vi "VM_ProjetoV5.2.vi"() -> ()   [LabVIEW 2016, in "Projeto_Modbus_Finalizado.lvlib"]
uses:
  <vilib>/userdefined/High Color/IMAQdx.ctl
  <vilib>/Analysis/baseanly.llb/Mean (DBL).vi
  <vilib>/lvdsc/process/Deploy Library.vi
  <vilib>/Utility/file.llb/Read Delimited Spreadsheet (DBL).vi
  <vilib>/Utility/file.llb/Write Delimited Spreadsheet (DBL).vi
  <vilib>/lvdsc/process/Undeploy Library.vi
  Projeto_Modbus_Finalizado.lvlib
  <vilib>/vision/driver/NI_Vision_Acquisition_Software.lvlib
  <resource>/objmgr/imaqdx.rc
  <vilib>/Analysis/NI_AALBase.lvlib
  <vilib>/lvdsc/NI_DSC.lvlib
panel:
  in  "Calibração\nRobô":path=path "C:/Users/rodrigorg1/Desktop/Projeto/calibracaoRobo.csv"
  in  "Calibração\nMesa":path=path "C:/Users/rodrigorg1/Desktop/Projeto/calibracaoMesa.csv"
  out "Error Out":errorcluster
  in  "Cut Limit":dbl=55.0 format="%#_13g"
  in  "Confirma":bool
  out "Status":string
  out "Câmera Robo":T1(plugin-control)
  out "Câmera Mesa":T1(plugin-control)
  in  "Começa jogada":bool
  in  "stop":bool
  in  "Source Câmera Robo":T2="S1156978"
  in  "Source Câmera Mesa":T2="cam0"
  out "Dobrao":bool
  out "Passa Vez":bool
  out "place pos Norm":dbl[](array[numeric])
  out "pick pos Norm":dbl[](array[numeric])
  out "place angle":dbl
  out "pick angle":dbl
  # "x 91\ny 176"
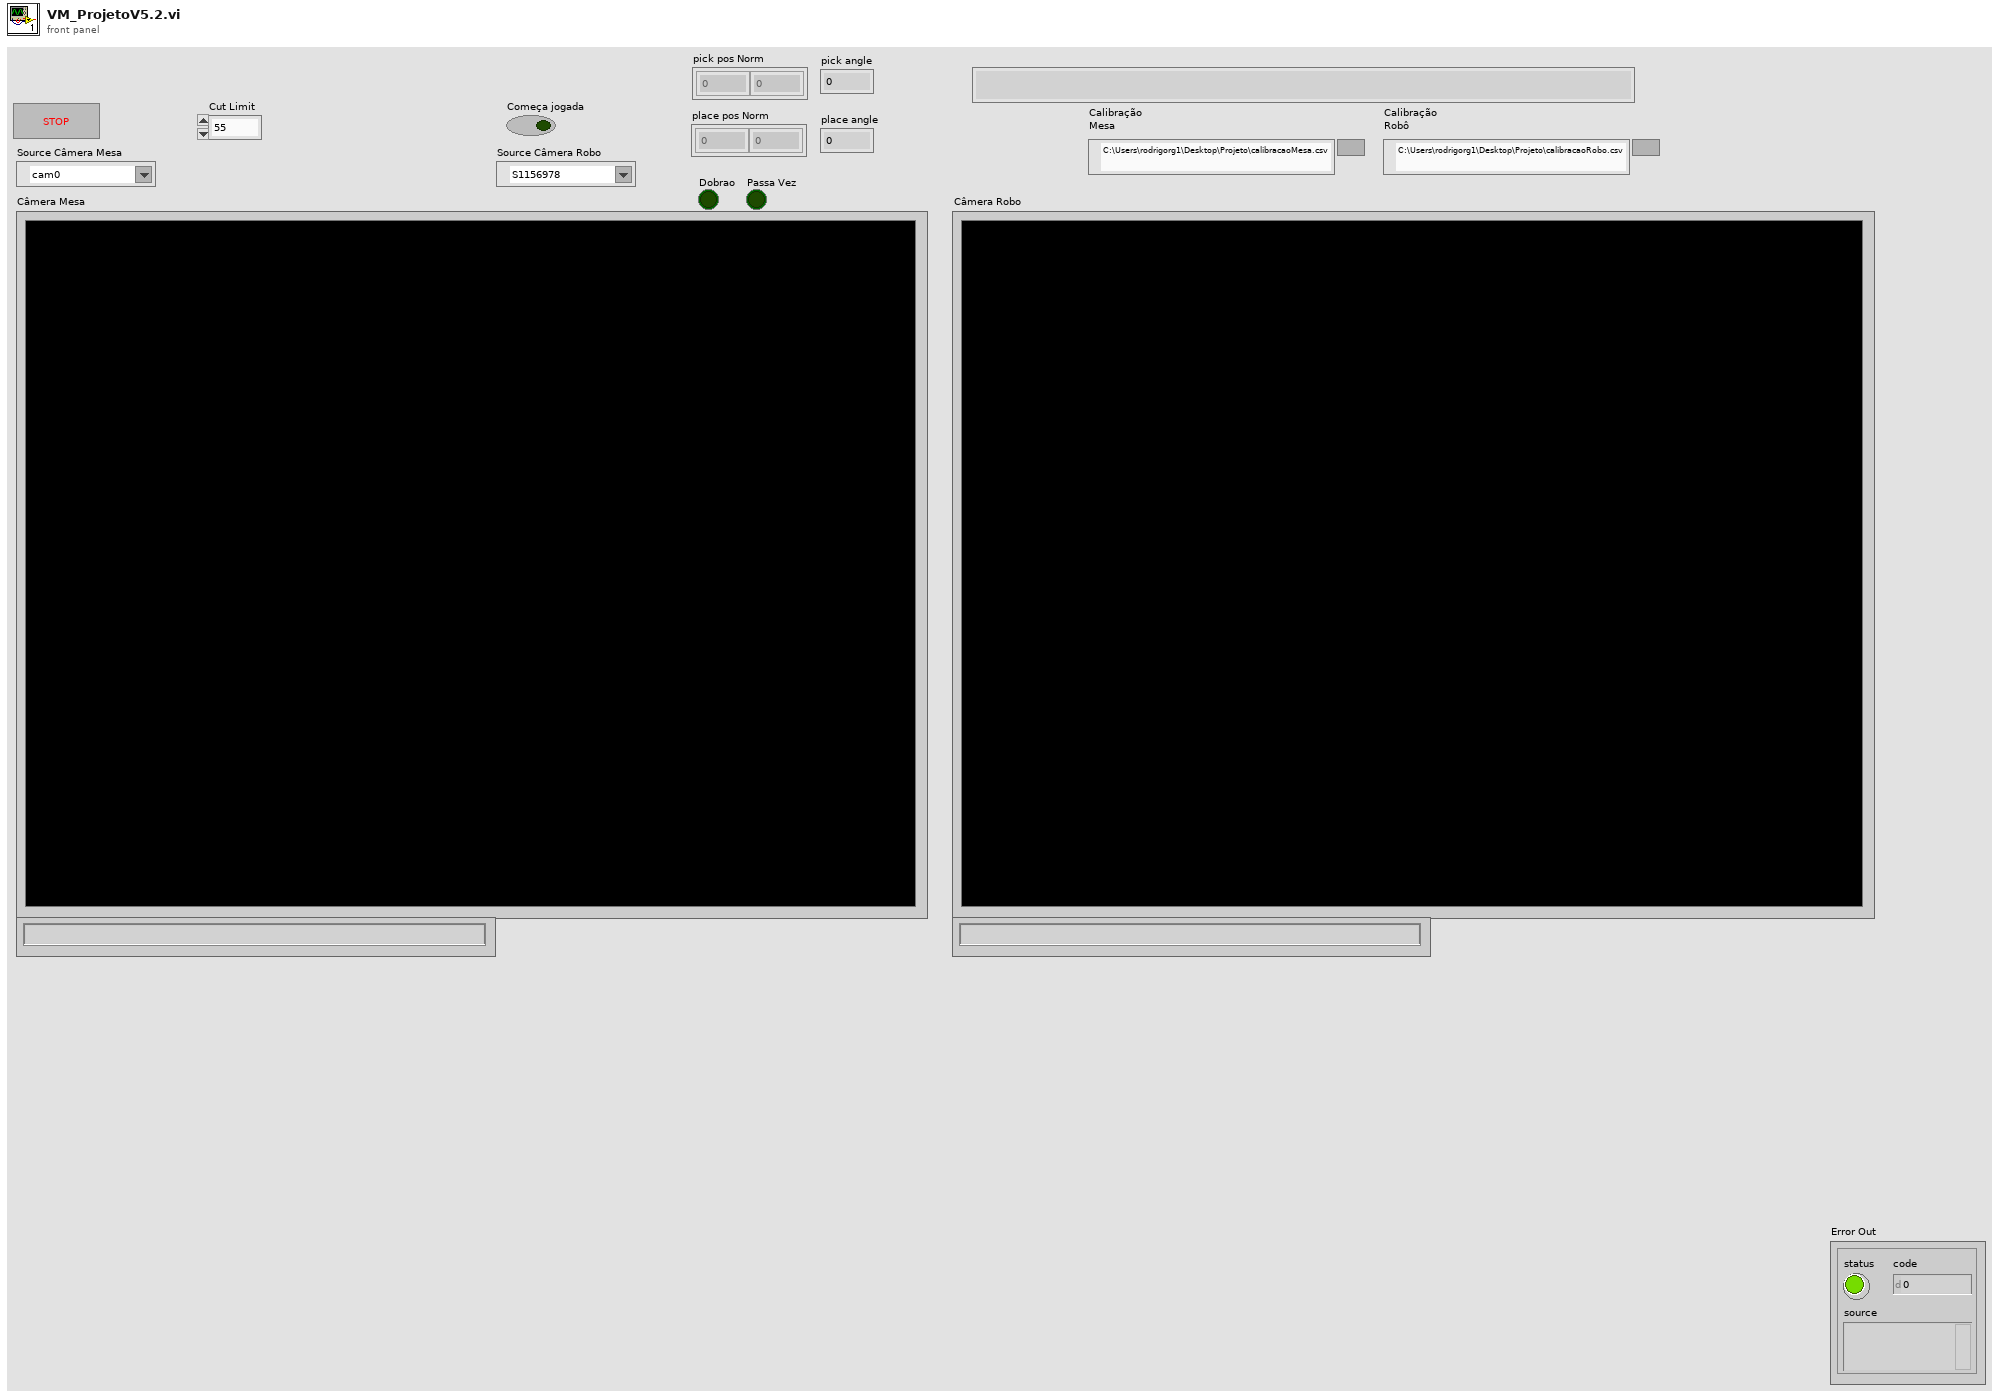
[diagram p1: front panel]
types:
  T1 = typedef "IMAQ Image.ctl" = refnum<image>
  T2 = typedef "IMAQdx.ctl" = refnum<k21>
  T3 = typedef "IMAQ Rectangle" = cluster{"Left":i32, "Top":i32, "Right":i32, "Bottom":i32, "Rotation":dbl}
  T4 = typedef "ROI Descriptor" = cluster{"Global Rectangle":i32[], "Contours":cluster{"ID":enum32{"External", "Internal"}, "Type":u32, "Coordinates":i32[]}[]}
  T5 = cluster{"Position":cluster{"x":sgl, "y":sgl}, "Angle":sgl, "Scale":sgl, "Score":sgl, "Bounding Box":cluster{"x":sgl, "y":sgl}[]}[]
  T6 = cluster{"Centro Peça":dbl[], "Centros Númeors":dbl[][], "Números":u8[], "ROI Números":T4[]}[]
  T7 = cluster{"Centro Peça":dbl[], "Centros Númeors":dbl[][], "Números":u8[], "ROI Números":T4[]}
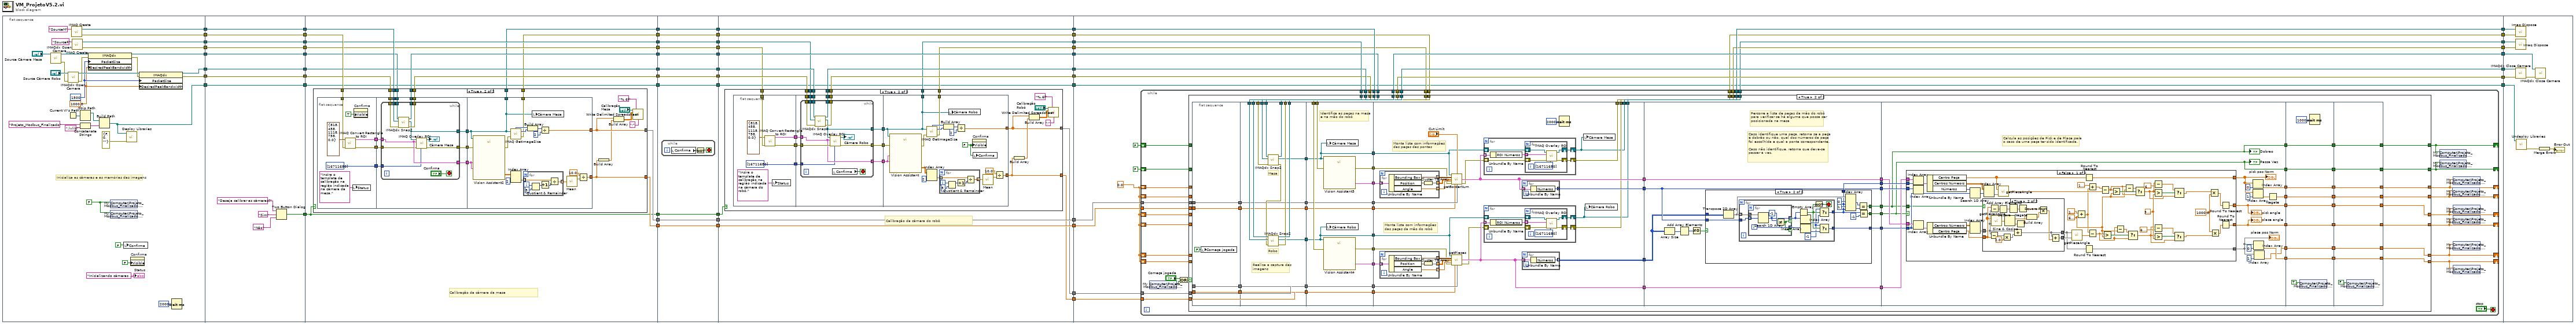
[diagram p0: block diagram]
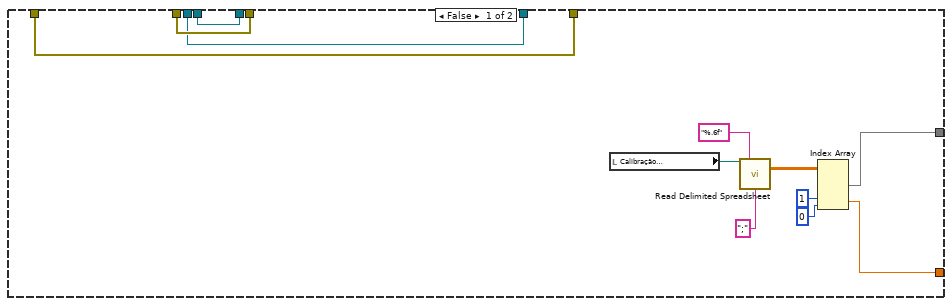
[diagram p2: hidden frame]
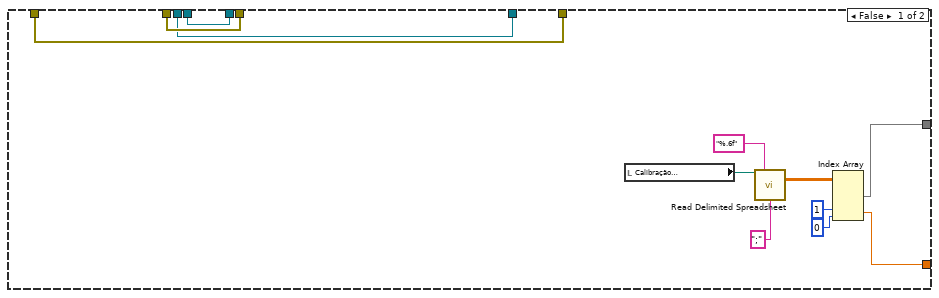
[diagram p3: hidden frame]
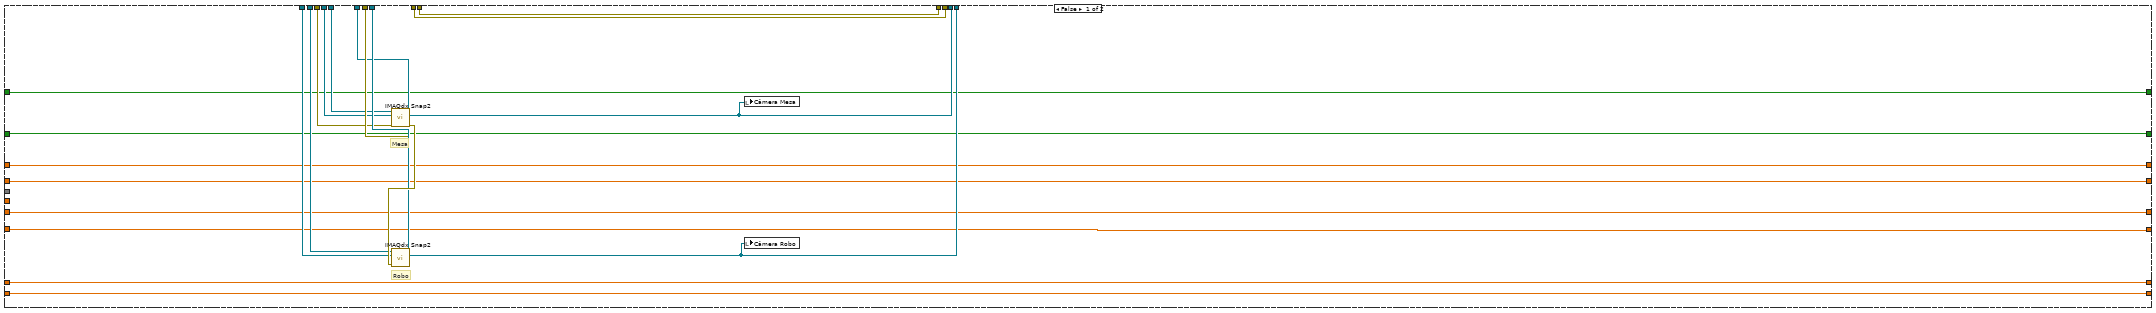
[diagram p4: hidden frame]
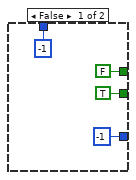
[diagram p5: hidden frame]
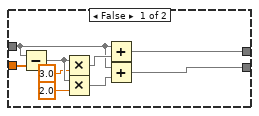
[diagram p6: hidden frame]
diagram:
  n1 = flat-sequence {
    tunnel: [w85] -> w17
    tunnel: [w84] -> w15
    tunnel: [w79] -> w13
    tunnel: [w83] -> w11
    tunnel: [w82] -> w9
    tunnel: [w78] -> w7
    tunnel: [w69] -> w5
    tunnel: [w61] -> w3
    tunnel: w17 -> [w101]
    tunnel: [w101] -> w16
    tunnel: w15 -> [w100]
    tunnel: [w100] -> w14
    tunnel: w13 -> [w99]
    tunnel: [w99] -> w12
    tunnel: w11 -> [w98]
    tunnel: [w98] -> w10
    tunnel: w9 -> [w97]
    tunnel: [w97] -> w8
    tunnel: w7 -> [w96]
    tunnel: [w96] -> w6
    tunnel: w5 -> [w95]
    tunnel: [w95] -> w4
    tunnel: w3 -> [w94]
    tunnel: [w94] -> w2
    tunnel: [w90] -> w1
    tunnel: w16 -> [w115]
    tunnel: w14 -> [w116]
    tunnel: w12 -> [w105]
    tunnel: w10 -> [w114]
    tunnel: w8 -> [w113]
    tunnel: w6 -> [w104]
    tunnel: [w109] -> w41
    tunnel: [w108] -> w39
    tunnel: [w114] -> w37
    tunnel: [w113] -> w35
    tunnel: [w112] -> w33
    tunnel: [w111] -> w31
    tunnel: w4 -> [w111]
    tunnel: [w110] -> w29
    tunnel: [w107] -> w27
    tunnel: [w106] -> w25
    tunnel: [w103] -> w20
    tunnel: w2 -> [w103]
    tunnel: [w102] -> w19
    tunnel: w1 -> [w102]
    tunnel: w41 -> [w213]
    tunnel: [w213] -> w40
    tunnel: w39 -> [w212]
    tunnel: [w212] -> w38
    tunnel: w37 -> [w211]
    tunnel: [w211] -> w36
    tunnel: w35 -> [w210]
    tunnel: [w210] -> w34
    tunnel: w33 -> [w209]
    tunnel: [w209] -> w32
    tunnel: w31 -> [w208]
    tunnel: [w208] -> w30
    tunnel: w29 -> [w207]
    tunnel: [w207] -> w28
    tunnel: w27 -> [w206]
    tunnel: [w206] -> w26
    tunnel: w25 -> [w205]
    tunnel: [w205] -> w24
    tunnel: [w204] -> w21
    tunnel: w20 -> [w204]
    tunnel: w19 -> [w203]
    tunnel: [w203] -> w18
    tunnel: w40 -> [w232]
    tunnel: [w232] -> w52
    tunnel: w38 -> [w231]
    tunnel: [w231] -> w51
    tunnel: w36 -> [w223]
    tunnel: [w222] -> w50
    tunnel: w34 -> [w221]
    tunnel: [w220] -> w49
    tunnel: w32 -> [w230]
    tunnel: [w230] -> w48
    tunnel: w30 -> [w225]
    tunnel: [w224] -> w47
    tunnel: w28 -> [w227]
    tunnel: [w226] -> w46
    tunnel: w26 -> [w229]
    tunnel: [w229] -> w45
    tunnel: w24 -> [w228]
    tunnel: [w228] -> w44
    tunnel: [w219] -> w43
    tunnel: [w218] -> w42
    tunnel: [w217] -> w22
    tunnel: w21 -> [w217]
    tunnel: w18 -> [w216]
    tunnel: [w337] -> w59
    tunnel: [w340] -> w58
    tunnel: [w334] -> w57
    tunnel: [w339] -> w56
    tunnel: [w338] -> w55
    tunnel: [w336] -> w54
    tunnel: [w335] -> w53
    tunnel: w52 -> [w333]
    tunnel: w51 -> [w332]
    tunnel: w50 -> [w331]
    tunnel: w49 -> [w330]
    tunnel: w48 -> [w329]
    tunnel: w47 -> [w328]
    tunnel: w46 -> [w327]
    tunnel: w45 -> [w325]
    tunnel: w44 -> [w326]
    tunnel: w43 -> [w323]
    tunnel: w42 -> [w324]
    tunnel: [w322] -> w23
    tunnel: w22 -> [w322]
    tunnel: w59 -> [w735]
    tunnel: w58 -> [w733]
    tunnel: w57 -> [w737]
    tunnel: w56 -> [w740]
    tunnel: w55 -> [w739]
    tunnel: w54 -> [w736]
    tunnel: w53 -> [w738]
    tunnel: w23 -> [w730]
    frame #0 {
      w60 = FALSE ("000021")
      w73 = 1000.0 ("DesiredPeakBandwidth")
      w74 = u32 1500 ("PacketSize")
      # "Inicializa as câmeras e as memórias das imagens"
      n2 = call <vilib>:"IMAQdx Open Camera.vi"("Session In"="Source Câmera Mesa") -> ("error out"=w77:errorcluster, "Session Out"=w80:T2)  [unwired: 9 in]
      n3 = Current VI's Path() -> (path=w62:path)
      n4 = call <vilib>:"IMAQdx Open Camera.vi"("error in"=w77, "Session In"="Source Câmera Robo") -> ("error out"=w76:errorcluster, "Session Out"=w81:T2)  [unwired: 8 in]
      n5 = call "IMAQ Create"("Image Name"="SourceM") -> ("New Image"=w85:T1, "error out"=w84:errorcluster)  [unwired: 4 in]
      n6 = call "IMAQ Create"("Image Name"="SourceR") -> ("New Image"=w83:T1, "error out"=w82:errorcluster)  [unwired: 4 in]
      n7 = Strip Path(path=w62) -> (stripped path=w63:path)  [unwired: 1 out]
      n8 = Concatenate Strings("Projeto_Modbus_Finalizado" ("library path"), ".lvlib" ("string")) -> (w66:string)
      n9 = property class="IMAQdx"(reference=w80, error in=w76, "PacketSize"=w74, "DesiredPeakBandwidth"=w73) -> (reference out=w79:T2, error out=w75:errorcluster)
      n10 = Build Path(base path=w63, name or relative path=w66) -> (appended path=w61:path)
      n11 = shared-variable "My Computer\\Projeto_Modbus_Finalizado.lvlib\\000021"(w60) -> ()  [unwired: 1 in, 1 out]
      n12 = shared-variable "My Computer\\Projeto_Modbus_Finalizado.lvlib\\000020"(w60) -> ()  [unwired: 1 in, 1 out]
      n13 = local write "Confirma"(FALSE ("Confirma")) -> ()
      n14 = call-poly <vilib>:"Deploy Libraries.vi"("error in (no error)"=errorcluster {"status"=FALSE, "code"=0, "source"=""}, "library path"=w61) -> ()  [unwired: 7 in, 1 out]
      n15 = property on="Confirma" class="Bool (strict)"("Visible"=FALSE) -> ()  [unwired: 2 in, 2 out]
      n16 = property class="IMAQdx"(reference=w81, error in=w75, "PacketSize"=w74, "DesiredPeakBandwidth"=w73) -> (reference out=w69:T2, error out=w78:errorcluster)
      n17 = Wait (ms)(milliseconds to wait=u32 2000) -> ()  [unwired: 1 out]
      "Status" <- "Inicializando câmeras ..." ("Status")
    }
    frame #1 {
      n18 = Two Button Dialog(message="Deseja calibrar as câmeras?", 1:"Não" ("F button name (\"Cancel\")"), 2:"Sim" ("T button name (\"OK\")")) -> (T button?=w90:bool)
    }
    frame #2 {
      # "Calibração da câmera da mesa"
      n19 = case shown="True" w102 {
        tunnel: w116 -> [w125 w143]
        tunnel: w115 -> [w126 w142]
        tunnel: [w127 w141] -> w112
        tunnel: [w128 w140] -> w110
        tunnel: [w126 w139] -> w109
        tunnel: [w125 w138] -> w108
        tunnel: [w118 w133] -> w107
        tunnel: [w117 w134] -> w106
        tunnel: w105 -> [w127 w137]
        tunnel: w104 -> [w128 w136]
        frame False {
          n20 = local read "Calibração\nMesa"() -> (w124:path)
          n21 = call-poly <vilib>:"Read Delimited Spreadsheet.vi"("file path (dialog if empty)"=w124, "format (%.3f)"="%.6f", "delimiter (\\t)"=";" ("delimiter (\\t)")) -> ("all rows"=w121:dbl[][])  [unwired: 7 in, 5 out]
          n22 = Index Array(array=w121, index (row) #2=1, index (col) #2=0) -> (element #1=w117:dbl[], element #2=w118:dbl)  [unwired: 2 in]
        }
        frame True {
          n23 = flat-sequence {
            tunnel: w143 -> [w154]
            tunnel: [w152] -> w149
            tunnel: [w151] -> w148
            tunnel: [u32[] [16711680] ("Colors (Green)")] -> w147
            tunnel: w137 -> [w167]
            tunnel: w136 -> [w166]
            tunnel: w142 -> [w165]
            tunnel: [w164] -> w141
            tunnel: [w163] -> w140
            tunnel: w149 -> [w162]
            tunnel: w148 -> [w161]
            tunnel: [w160] -> w146
            tunnel: [w159] -> w145
            tunnel: [w158] -> w144
            tunnel: w147 -> [w157]
            tunnel: w146 -> [w196]
            tunnel: w145 -> [w195]
            tunnel: [w187] -> w133
            tunnel: w144 -> [w180]
            tunnel: [w180] -> w139
            tunnel: [w182] -> w138
            tunnel: [w181] -> w134
            frame #0 {
              n24 = call "IMAQ Convert Rectangle to ROI"("error in (no error)"=w154, "Rectangle"=T3 {"Left"=818, "Top"=458, "Right"=1118, "Bottom"=758, "Rotation"=0.0}) -> ("error out"=w152:errorcluster, "ROI Descriptor"=w151:T4)  [unwired: 7 in]
              n25 = local write "Status"("Insira o template de calibração na região indicada na câmera da mesa." ("Status")) -> ()
              n26 = property on="Confirma" class="Bool (strict)"("Visible"=TRUE) -> ()  [unwired: 2 in, 2 out]
            }
            frame #1 {
              n27 = while {
                tunnel: w167 -> [w178]
                tunnel: w166 -> [w177]
                tunnel: w165 -> [w176]
                tunnel: [w175] -> w164
                tunnel: [w174] -> w163
                tunnel: w162 -> [w168]
                tunnel: w161 -> [w171]
                tunnel: [w173] -> w160
                tunnel: [w171] -> w159
                tunnel: [w169] -> w158
                tunnel: w157 -> [w170]
                stop <- "Confirma" stop-if-true
                n28 = call <vilib>:"IMAQdx Snap2.vi"("error in"=w177, "Image In"=w176, "Session In"=w178) -> ("error out"=w174:errorcluster, "Image Out"=w169:T1, "Session Out"=w175:T2)  [unwired: 6 in]
                n29 = call "IMAQ Overlay ROI"("Colors (Green)"=w170, "error in (no error)"=w168, "ROI Descriptor"=w171, "Image"=w169) -> ("error out"=w173:errorcluster, "Image Out"=→"Câmera Mesa":T1)  [unwired: 6 in]
              }
            }
            frame #2 {
              n30 = call "Vision Assistant2"("Image In"=w180, "ROI Descriptor (Adv. Straight Edge 1)"=w195, "ROI Descriptor (Copy of Adv. Straight Edge 1)"=w195, "error in"=w196) -> ("Caliper Results (Caliper 2)"=w194:sgl[][], "error out"=w188:errorcluster)  [unwired: 21 in, 1 out]
              n31 = call "IMAQ GetImageSize"("Image"=w180, "error in (no error)"=w188) -> ("Y Resolution"=w186:i32, "X Resolution"=w185:i32, "error out"=w182:errorcluster)  [unwired: 2 in]
              n32 = Index Array(array=w194, index (col)=2 ("disabled index (col)")) -> (element=w192:sgl[])  [unwired: 1 in]
              n33 = for {
                tunnel: w192 -> [w199] mode=indexing
                tunnel: [w197] -> w191 mode=indexing
                i -> [w202]
                n34 = Quotient & Remainder(x=w202, y=5) -> (x-y*floor(x/y)=w200:i32)  [unwired: 1 out]
                n35 = Increment(x=w200) -> (x+1=w198:i32)
                n36 = Divide(x=w199, y=w198) -> (x/y=w197:sgl)
              }
              n37 = Build Array(w185, w186) -> (w184:i32[])
              n38 = local write "Câmera Mesa"(w180) -> ()
              n39 = Divide(x=w184, y=2) -> (x/y=w181:dbl[])
              n40 = call-poly <vilib>:"Mean.vi"("X"=w191) -> ("mean"=w190:dbl)  [unwired: 1 out]
              n41 = Divide(x=10.0, y=w190) -> (x/y=w187:dbl)
            }
          }
          n42 = Build Array(w133) -> (w132:dbl[])
          n43 = Build Array(w134, w132) -> (w131:dbl[][])
          n44 = call-poly <vilib>:"Write Delimited Spreadsheet.vi"("file path (dialog if empty)"="Calibração\nMesa", "format (%.3f)"="%.6f", "2D data"=w131, "delimiter (\\t)"=";" ("delimiter (\\t)")) -> ()  [unwired: 10 in, 2 out]
        }
      }
    }
    frame #3 {
      n45 = while {
        stop <- w215 stop-if-true
        n46 = local read "Confirma"() -> (w214:bool)
        n47 = Not(x=w214) -> (.not. x?=w215:bool)
      }
    }
    frame #4 {
      # "Calibração da câmera do robô"
      n48 = case shown="True" w216 {
        tunnel: w227 -> [w243 w259]
        tunnel: [w243 w258] -> w226
        tunnel: w225 -> [w244 w257]
        tunnel: [w244 w256] -> w224
        tunnel: w223 -> [w242 w255]
        tunnel: [w242 w254] -> w222
        tunnel: w221 -> [w241 w253]
        tunnel: [w241 w252] -> w220
        tunnel: [w233 w246] -> w219
        tunnel: [w234 w245] -> w218
        frame False {
          n49 = local read "Calibração\nRobô"() -> (w235:path)
          n50 = call-poly <vilib>:"Read Delimited Spreadsheet.vi"("file path (dialog if empty)"=w235, "format (%.3f)"="%.6f", "delimiter (\\t)"=";" ("delimiter (\\t)")) -> ("all rows"=w238:dbl[][])  [unwired: 7 in, 5 out]
          n51 = Index Array(array=w238, index (row) #2=1, index (col) #2=0) -> (element #1=w234:dbl[], element #2=w233:dbl)  [unwired: 2 in]
        }
        frame True {
          n52 = flat-sequence {
            tunnel: w253 -> [w270]
            tunnel: [w269] -> w265
            tunnel: [w268] -> w264
            tunnel: [u32[] [16711680] ("Colors (Green)")] -> w263
            tunnel: w257 -> [w282]
            tunnel: w259 -> [w281]
            tunnel: w255 -> [w280]
            tunnel: [w279] -> w256
            tunnel: [w278] -> w258
            tunnel: w265 -> [w277]
            tunnel: w264 -> [w276]
            tunnel: [w275] -> w262
            tunnel: [w274] -> w261
            tunnel: [w273] -> w260
            tunnel: w263 -> [w272]
            tunnel: w262 -> [w312]
            tunnel: w261 -> [w311]
            tunnel: [w303] -> w246
            tunnel: w260 -> [w296]
            tunnel: [w296] -> w254
            tunnel: [w298] -> w252
            tunnel: [w297] -> w245
            frame #0 {
              n53 = call "IMAQ Convert Rectangle to ROI"("error in (no error)"=w270, "Rectangle"=T3 {"Left"=818, "Top"=458, "Right"=1118, "Bottom"=758, "Rotation"=0.0}) -> ("error out"=w269:errorcluster, "ROI Descriptor"=w268:T4)  [unwired: 7 in]
              n54 = local write "Status"("Insira o template de calibração na região indicada na câmera do robô." ("Status")) -> ()
            }
            frame #1 {
              n55 = while {
                tunnel: w282 -> [w294]
                tunnel: w281 -> [w293]
                tunnel: w280 -> [w292]
                tunnel: [w291] -> w279
                tunnel: [w290] -> w278
                tunnel: w277 -> [w289]
                tunnel: w276 -> [w287]
                tunnel: [w288] -> w275
                tunnel: [w287] -> w274
                tunnel: [w286] -> w273
                tunnel: w272 -> [w285]
                stop <- w283 stop-if-true
                n56 = call <vilib>:"IMAQdx Snap2.vi"("error in"=w293, "Image In"=w292, "Session In"=w294) -> ("error out"=w290:errorcluster, "Image Out"=w286:T1, "Session Out"=w291:T2)  [unwired: 6 in]
                n57 = call "IMAQ Overlay ROI"("Colors (Green)"=w285, "error in (no error)"=w289, "ROI Descriptor"=w287, "Image"=w286) -> ("error out"=w288:errorcluster, "Image Out"=→"Câmera Robo":T1)  [unwired: 6 in]
                n58 = local read "Confirma"() -> (w283:bool)
              }
            }
            frame #2 {
              w295 = FALSE ("Visible")
              n59 = call "Vision Assistant"("Image In"=w296, "ROI Descriptor (Adv. Straight Edge 1)"=w311, "ROI Descriptor (Copy of Adv. Straight Edge 1)"=w311, "error in"=w312) -> ("Caliper Results (Caliper 2)"=w310:sgl[][], "error out"=w304:errorcluster)  [unwired: 21 in, 1 out]
              n60 = call "IMAQ GetImageSize"("Image"=w296, "error in (no error)"=w304) -> ("Y Resolution"=w302:i32, "X Resolution"=w301:i32, "error out"=w298:errorcluster)  [unwired: 2 in]
              n61 = Index Array(array=w310, index (col)=2 ("disabled index (col)")) -> (element=w308:sgl[])  [unwired: 1 in]
              n62 = for {
                tunnel: w308 -> [w315] mode=indexing
                tunnel: [w313] -> w307 mode=indexing
                i -> [w318]
                n63 = Quotient & Remainder(x=w318, y=5) -> (x-y*floor(x/y)=w316:i32)  [unwired: 1 out]
                n64 = Increment(x=w316) -> (x+1=w314:i32)
                n65 = Divide(x=w315, y=w314) -> (x/y=w313:sgl)
              }
              n66 = Build Array(w301, w302) -> (w300:i32[])
              n67 = local write "Câmera Robo"(w296) -> ()
              n68 = Divide(x=w300, y=2) -> (x/y=w297:dbl[])
              n69 = property on="Confirma" class="Bool (strict)"("Visible"=w295) -> ()  [unwired: 2 in, 2 out]
              n70 = local write "Confirma"(w295) -> ()
              n71 = call-poly <vilib>:"Mean.vi"("X"=w307) -> ("mean"=w306:dbl)  [unwired: 1 out]
              n72 = Divide(x=10.0, y=w306) -> (x/y=w303:dbl)
            }
          }
          n73 = Build Array(w246) -> (w250:dbl[])
          n74 = Build Array(w245, w250) -> (w249:dbl[][])
          n75 = call-poly <vilib>:"Write Delimited Spreadsheet.vi"("file path (dialog if empty)"="Calibração\nRobô", "format (%.3f)"="%.6f", "2D data"=w249, "delimiter (\\t)"=";" ("delimiter (\\t)")) -> ()  [unwired: 10 in, 2 out]
        }
      }
    }
    frame #5 {
      w319 = 0.0 ("Numeric")
      n76 = while {
        tunnel: w329 -> [w378]
        tunnel: w333 -> [w377]
        tunnel: w331 -> [w376]
        tunnel: w328 -> [w375]
        tunnel: w327 -> [w374]
        tunnel: [w373] -> w340
        tunnel: [w372] -> w339
        tunnel: [w371] -> w338
        tunnel: w332 -> [w370]
        tunnel: w330 -> [w369]
        tunnel: [w368] -> w337
        tunnel: [w367] -> w334
        tunnel: [w365] -> w336
        tunnel: [w364] -> w335
        tunnel: w326 -> [w363]
        tunnel: w325 -> [w362]
        tunnel: w324 -> [w361]
        tunnel: w323 -> [w360]
        shift-right: [w356] -> _
        shift-left: FALSE -> [w347]
        shift-right: [w355] -> _
        shift-left: FALSE -> [w348]
        shift-right: [w354] -> _
        shift-left: w319 -> [w346]
        shift-right: [w353] -> _
        shift-left: w319 -> [w345]
        shift-right: [w352] -> _
        shift-left: w319 -> [w344]
        shift-right: [w351] -> _
        shift-left: w319 -> [w343]
        shift-right: [w350] -> _
        shift-left: w319 -> [w342]
        shift-right: [w349] -> _
        shift-left: w319 -> [w341]
        stop <- "stop" stop-if-true
        n77 = shared-variable "My Computer\\Projeto_Modbus_Finalizado.lvlib\\000022"() -> (w357:bool)  [unwired: 1 in, 1 out]
        n78 = Or(x="Começa jogada", y=w357) -> (x .or. y?=w359:bool)
        n79 = case shown="True" w359 {
          tunnel: w378 -> [w390 w472]
          tunnel: w377 -> [w389 w471]
          tunnel: w376 -> [w396 w470]
          tunnel: w375 -> [w395 w469]
          tunnel: w374 -> [w392 w468]
          tunnel: [w391 w467] -> w373
          tunnel: [w394 w466] -> w372
          tunnel: [w393 w465] -> w371
          tunnel: w370 -> [w399 w463]
          tunnel: w369 -> [w398 w461]
          tunnel: [w388 w429] -> w368
          tunnel: [w387 w430] -> w367
          tunnel: [w399 w427] -> w365
          tunnel: [w398 w428] -> w364
          tunnel: w363 -> [_ w416]
          tunnel: w362 -> [_ w443]
          tunnel: w361 -> [_ w418]
          tunnel: w360 -> [_ w417]
          tunnel: [w384 w426] -> w354
          tunnel: [w382 w425] -> w353
          tunnel: [w383 w424] -> w352
          tunnel: [w381 w423] -> w351
          tunnel: [w380 w422] -> w350
          tunnel: [w379 w421] -> w349
          tunnel: [w385 w420] -> w356
          tunnel: [w386 w419] -> w355
          tunnel: w348 -> [w386 _]
          tunnel: w347 -> [w385 _]
          tunnel: w346 -> [w384 _]
          tunnel: w345 -> [w382 _]
          tunnel: w344 -> [w383 _]
          tunnel: w343 -> [w381 _]
          tunnel: w342 -> [w380 _]
          tunnel: w341 -> [w379 _]
          frame False {
            # "Robo"
            # "Mesa"
            n80 = call <vilib>:"IMAQdx Snap2.vi"("error in"=w392, "Image In"=w389, "Session In"=w390) -> ("error out"=w397:errorcluster, "Image Out"=w388:T1, "Session Out"=w391:T2)  [unwired: 6 in]
            n81 = call <vilib>:"IMAQdx Snap2.vi"("error in"=w397, "Image In"=w396, "Session In"=w395) -> ("error out"=w393:errorcluster, "Image Out"=w387:T1, "Session Out"=w394:T2)  [unwired: 6 in]
            n82 = local write "Câmera Mesa"(w388) -> ()
            n83 = local write "Câmera Robo"(w387) -> ()
          }
          frame True {
            n84 = flat-sequence {
              tunnel: w417 -> [w474]
              tunnel: w418 -> [w475]
              tunnel: w443 -> [w476]
              tunnel: w416 -> [w477]
              tunnel: [w477] -> w434
              tunnel: [w476] -> w433
              tunnel: [w475] -> w432
              tunnel: [w474] -> w431
              tunnel: w472 -> [w492]
              tunnel: w471 -> [w491]
              tunnel: w470 -> [w490]
              tunnel: w469 -> [w489]
              tunnel: w468 -> [w483]
              tunnel: [w488] -> w467
              tunnel: [w487] -> w466
              tunnel: [w486] -> w465
              tunnel: [w485] -> w464
              tunnel: [w484] -> w462
              tunnel: [w481] -> w441
              tunnel: [w480] -> w439
              tunnel: [w479] -> w437
              tunnel: [w478] -> w436
              tunnel: w434 -> [w481]
              tunnel: w433 -> [w480]
              tunnel: w432 -> [w479]
              tunnel: w431 -> [w478]
              tunnel: w464 -> [w494]
              tunnel: w463 -> [w504]
              tunnel: w462 -> [w493]
              tunnel: w461 -> [w503]
              tunnel: [w502] -> w460
              tunnel: [w501] -> w459
              tunnel: [w493] -> w458
              tunnel: [w494] -> w457
              tunnel: [w500] -> w456
              tunnel: [w499] -> w455
              tunnel: [w498] -> w442
              tunnel: w441 -> [w498]
              tunnel: [w497] -> w440
              tunnel: w439 -> [w497]
              tunnel: [w496] -> w438
              tunnel: w437 -> [w496]
              tunnel: w436 -> [w495]
              tunnel: [w495] -> w435
              tunnel: w460 -> [w532]
              tunnel: w459 -> [w531]
              tunnel: w458 -> [w506]
              tunnel: w457 -> [w507]
              tunnel: w456 -> [w527]
              tunnel: w455 -> [w523]
              tunnel: [w522] -> w454
              tunnel: [w521] -> w453
              tunnel: [w515] -> w452
              tunnel: [w513] -> w451
              tunnel: w442 -> [w520]
              tunnel: w440 -> [w519]
              tunnel: w438 -> [w518]
              tunnel: w435 -> [w517]
              tunnel: [w508] -> w430
              tunnel: [w511] -> w428
              tunnel: [w509] -> w429
              tunnel: [w510] -> w427
              tunnel: w454 -> [w575]
              tunnel: w453 -> [w574]
              tunnel: w452 -> [w581]
              tunnel: w451 -> [w577]
              tunnel: [w581] -> w450
              tunnel: [w580] -> w449
              tunnel: [w579] -> w448
              tunnel: [w578] -> w447
              tunnel: [w577] -> w446
              tunnel: [w576] -> w445
              tunnel: [w575] -> w444
              tunnel: w450 -> [w631]
              tunnel: w449 -> [w621]
              tunnel: w448 -> [w622]
              tunnel: w447 -> [w634]
              tunnel: w446 -> [w630]
              tunnel: w445 -> [w633]
              tunnel: w444 -> [w632]
              tunnel: [w623] -> w415
              tunnel: [w615] -> w414
              tunnel: [w620] -> w413
              tunnel: [w619] -> w412
              tunnel: [w617] -> w411
              tunnel: [w618] -> w410
              tunnel: [w622] -> w409
              tunnel: [w621] -> w408
              tunnel: w415 -> [w720]
              tunnel: w414 -> [w719]
              tunnel: w413 -> [w718]
              tunnel: w412 -> [w717]
              tunnel: w411 -> [w716]
              tunnel: w410 -> [w715]
              tunnel: w409 -> [w714]
              tunnel: w408 -> [w713]
              tunnel: [w720] -> w407
              tunnel: [w719] -> w406
              tunnel: [w718] -> w405
              tunnel: [w717] -> w404
              tunnel: [w716] -> w403
              tunnel: [w715] -> w402
              tunnel: [w714] -> w401
              tunnel: [w713] -> w400
              tunnel: [w722] -> w419
              tunnel: [w723] -> w420
              tunnel: [w724] -> w421
              tunnel: [w725] -> w422
              tunnel: [w726] -> w423
              tunnel: [w727] -> w424
              tunnel: [w728] -> w425
              tunnel: [w729] -> w426
              tunnel: w407 -> [w729]
              tunnel: w406 -> [w728]
              tunnel: w405 -> [w727]
              tunnel: w404 -> [w726]
              tunnel: w403 -> [w725]
              tunnel: w402 -> [w724]
              tunnel: w401 -> [w723]
              tunnel: w400 -> [w722]
              frame #0 {
                n85 = local write "Começa jogada"(FALSE ("Começa jogada")) -> ()
              }
              frame #1 {
                # "Realiza a captura das\nimagens"
                # "Robo"
                # "Mesa"
                n86 = call <vilib>:"IMAQdx Snap2.vi"("error in"=w483, "Image In"=w491, "Session In"=w492) -> ("error out"=w482:errorcluster, "Image Out"=w485:T1, "Session Out"=w488:T2)  [unwired: 6 in]
                n87 = call <vilib>:"IMAQdx Snap2.vi"("error in"=w482, "Image In"=w490, "Session In"=w489) -> ("error out"=w486:errorcluster, "Image Out"=w484:T1, "Session Out"=w487:T2)  [unwired: 6 in]
              }
              frame #2 {
                # "Identifica as peças na mesa\ne na mão do robô"
                n88 = call "Vision Assistant3"("Image In"=w494, "error in"=w504) -> ("Matches (Pattern Matching 1)"=w501:T5, "error out"=w500:errorcluster)  [unwired: 23 in, 1 out]
                n89 = call "Vision Assistant4"("Image In"=w493, "error in"=w503) -> ("Matches (Pattern Matching 1)"=w502:T5, "error out"=w499:errorcluster)  [unwired: 23 in, 1 out]
                n90 = local write "Câmera Mesa"(w494) -> ()
                n91 = local write "Câmera Robo"(w493) -> ()
              }
              frame #3 {
                # "Monta lista com informações\ndas peças das pontas"
                # "Monta lista com informações\ndas peças da mão do robô"
                n92 = for {
                  tunnel: w531 -> [w565] mode=indexing
                  tunnel: [w563] -> w529 mode=indexing
                  tunnel: [w562] -> w530 mode=indexing
                  tunnel: [w561] -> w528 mode=indexing
                  n93 = Unbundle By Name(w565) -> ("Bounding Box"=w562:cluster{"x":sgl, "y":sgl}[], "Position"=w564:cluster{"x":sgl, "y":sgl}, "Angle"=w561:sgl)
                  n94 = Cluster To Array(cluster=w564) -> (array=w563:sgl[])
                }
                n95 = for {
                  tunnel: w532 -> [w570] mode=indexing
                  tunnel: [w568] -> w525 mode=indexing
                  tunnel: [w567] -> w526 mode=indexing
                  tunnel: [w566] -> w524 mode=indexing
                  n96 = Unbundle By Name(w570) -> ("Bounding Box"=w567:cluster{"x":sgl, "y":sgl}[], "Position"=w569:cluster{"x":sgl, "y":sgl}, "Angle"=w566:sgl)
                  n97 = Cluster To Array(cluster=w569) -> (array=w568:sgl[])
                }
                n98 = call "getBorderNum.vi"("Refnum in"=w507, "Cut Limit"="Cut Limit", "Bounding Box"=w530, "Position"=w529, "Angle"=w528, "error in (no error)"=w527, "Step"=w519, "Origin Pixel"=w520) -> ("Data Pieces"=w515:T6, "error out"=w514:errorcluster)  [unwired: 5 in, 1 out]
                n99 = call "getPieces.vi"("Refnum in"=w506, "Bounding Box"=w526, "Position"=w525, "Angle"=w524, "error in (no error)"=w523, "Step"=w517, "Origin Pixel"=w518) -> ("Data Pieces"=w513:T6, "error out"=w512:errorcluster)  [unwired: 6 in, 1 out]
                n100 = for {
                  tunnel: w515 -> [w550] mode=indexing
                  shift-right: [w547] -> w509
                  shift-left: w507 -> [w548]
                  shift-right: [w545] -> w510
                  shift-left: w514 -> [w546]
                  n101 = Unbundle By Name(w550) -> ("ROI Números"=w549:T4[])
                  n102 = for {
                    tunnel: w549 -> [w556] mode=indexing
                    shift-right: [w554] -> w547
                    shift-left: w548 -> [w555]
                    shift-right: [w552] -> w545
                    shift-left: w546 -> [w553]
                    n103 = call "IMAQ Overlay ROI"("Colors (Green)"=u32[] [16711680], "error in (no error)"=w553, "ROI Descriptor"=w556, "Image"=w555) -> ("error out"=w552:errorcluster, "Image Out"=w554:T1)  [unwired: 6 in]
                  }
                }
                n104 = for {
                  tunnel: w513 -> [w538] mode=indexing
                  shift-right: [w535] -> w508
                  shift-left: w506 -> [w536]
                  shift-right: [w533] -> w511
                  shift-left: w512 -> [w534]
                  n105 = Unbundle By Name(w538) -> ("ROI Números"=w537:T4[])
                  n106 = for {
                    tunnel: w537 -> [w544] mode=indexing
                    shift-right: [w542] -> w535
                    shift-left: w536 -> [w543]
                    shift-right: [w540] -> w533
                    shift-left: w534 -> [w541]
                    n107 = call "IMAQ Overlay ROI"("Colors (Green)"=u32[] [16711680], "error in (no error)"=w541, "ROI Descriptor"=w544, "Image"=w543) -> ("error out"=w540:errorcluster, "Image Out"=w542:T1)  [unwired: 6 in]
                  }
                }
                n108 = for {
                  tunnel: w515 -> [w560] mode=indexing
                  tunnel: [w559] -> w522 mode=concatenating
                  n109 = Unbundle By Name(w560) -> ("Números"=w559:u8[])
                }
                n110 = for {
                  tunnel: w513 -> [w558] mode=indexing
                  tunnel: [w557] -> w521 mode=indexing
                  n111 = Unbundle By Name(w558) -> ("Números"=w557:u8[])
                }
                n112 = Wait (ms)(milliseconds to wait=u32 2000) -> ()  [unwired: 1 out]
                n113 = local write "Câmera Mesa"(w509) -> ()
                n114 = local write "Câmera Robo"(w508) -> ()
              }
              frame #4 {
                # "Caso identifique uma peça, retorna se a peça\né dobrão ou não, qual dos números da peça\nfoi escolhida e qual a ponta correspondente.\n\nCaso não identifique, retorna que deve-se\npassar a vez."
                # "Percorre a lista de peças da mão do robô\npara verificar se há alguma que possa ser\nposicionada na mesa"
                n115 = Array Size(array=w574) -> (size(s)=w573:i32[])
                n116 = Add Array Elements(numeric array=w573) -> (sum=w572:i32)
                n117 = Not Equal To 0?(x=w572) -> (x != 0?=w571:bool)
                n118 = case shown="True" w571 {
                  tunnel: w574 -> [_ w591]
                  tunnel: [FALSE w590] -> w580
                  tunnel: [TRUE w589] -> w579
                  tunnel: [-1 ("t") w588] -> w578
                  tunnel: [-1 ("index of element") w587] -> w576
                  tunnel: w575 -> [_ w586]
                  frame False {
                  }
                  frame True {
                    n119 = Transpose 2D Array(2D array=w591) -> (transposed array=w593:u8[][])
                    n120 = for {
                      tunnel: w593 -> [w608] mode=indexing
                      tunnel: w586 -> [w607]
                      tunnel: [w599] -> w588
                      tunnel: [w598] -> w587
                      stop <- w603 stop-if-true
                      w600 = -1 ("t")
                      n121 = for {
                        tunnel: w608 -> [w614]
                        tunnel: w607 -> [w613] mode=indexing
                        tunnel: [w611] -> w605 mode=indexing if=w609
                        tunnel: [w610] -> w604 mode=indexing if=w609
                        i -> [w610]
                        n122 = Search 1D Array(1D array=w614, element=w613) -> (index of element=w611:i32)  [unwired: 1 in]
                        n123 = Not Equal?(x=w611, y=-1) -> (x != y?=w609:bool)
                      }
                      n124 = Empty Array?(array=w605) -> (empty?=w601:bool)
                      n125 = Index Array(array=w605) -> (element=w606:i32)  [unwired: 1 in]
                      n126 = Index Array(array=w604) -> (element=w602:i32)  [unwired: 1 in]
                      n127 = Not(x=w601) -> (.not. x?=w603:bool)
                      n128 = Select(t=w600, s=w601, f=w606) -> (s? t:f=w598:i32)
                      n129 = Select(t=w600, s=w601, f=w602) -> (s? t:f=w599:i32)
                    }
                    n130 = Index Array(array=w593, index (row) #1=0 ("disabled index (row)"), index (col) #1=w587, index (row) #2=1 ("disabled index (row)"), index (col) #2=w587) -> (element #1=w597:u8, element #2=w596:u8)
                    n131 = Equal?(x=w597, y=w596) -> (x = y?=w590:bool)
                    n132 = Equal?(x=w587, y=-1) -> (x = y?=w589:bool)
                  }
                }
              }
              frame #5 {
                # "Calcula as posições de Pick e de Place para\no caso de uma peça ter sido identificada."
                n133 = case shown="False" w622 {
                  tunnel: w630 -> [w680 _]
                  tunnel: w633 -> [w679 _]
                  tunnel: w634 -> [w676 _]
                  tunnel: w631 -> [w678 _]
                  tunnel: w632 -> [w668 _]
                  tunnel: w621 -> [w673 _]
                  tunnel: [w666 _] -> w628
                  tunnel: [w665 _] -> w624
                  tunnel: [w661 _] -> w619
                  tunnel: [w662 _] -> w620
                  frame False {
                    w645 = 3.141592653589793
                    w649 = 6.283185307179586
                    w667 = 1000.0
                    n134 = Index Array(array=w680, index=w679) -> (element=w681:T7)
                    n135 = Index Array(array=w668, index=w676) -> (element=w675:u8)
                    n136 = Index Array(array=w678, index=w676) -> (element=w677:T7)
                    n137 = Unbundle By Name(w681) -> ("Centro Peça"=w663:dbl[], "Centros Númeors"=w683:dbl[][], "Números"=w682:u8[])
                    n138 = Unbundle By Name(w677) -> ("Centros Númeors"=w670:dbl[][], "Centro Peça"=w669:dbl[])
                    n139 = Search 1D Array(1D array=w682, element=w675) -> (index of element=w684:i32)  [unwired: 1 in]
                    n140 = Index Array(array=w670) -> (element=w672:dbl[])  [unwired: 2 in]
                    n141 = case shown="True" w673 {
                      tunnel: w672 -> [w688 w703]
                      tunnel: w669 -> [w692 w704]
                      tunnel: [w686 w696] -> w671
                      tunnel: [w685 w695] -> w664
                      frame False {
                        n142 = Subtract(x=w688, y=w692) -> (x-y=w691:dbl[])
                        n143 = Multiply(x=w691, y=3.0) -> (x*y=w693:dbl[])
                        n144 = Multiply(x=w691, y=2.0) -> (x*y=w687:dbl[])
                        n145 = Add(x=w688, y=w693) -> (x+y=w685:dbl[])
                        n146 = Add(x=w688, y=w687) -> (x+y=w686:dbl[])
                      }
                      frame True {
                        n147 = Subtract(x=w703, y=w704) -> (x-y=w710:dbl[])
                        n148 = Subtract(x=w704, y=w703) -> (x-y=w707:dbl[])
                        n149 = call "getPieceAngle.vi"("Center Num"=w703, "Center Piece"=w704) -> ("Angle"=w702:dbl)
                        n150 = Square(x=w707) -> (x^2=w706:dbl[])
                        n151 = Multiply(x=w710, y=2.0) -> (x*y=w708:dbl[])
                        n152 = Sine & Cosine(0:w702) -> (1:w700:dbl, 2:w701:dbl)
                        n153 = Add Array Elements(numeric array=w706) -> (sum=w705:dbl)
                        n154 = Add(x=w703, y=w708) -> (x+y=w695:dbl[])
                        n155 = Negate(x=w701) -> (-x=w699:dbl)
                        n156 = Square Root(x=w705) -> (sqrt(x)=w697:dbl)
                        n157 = Build Array(w699, w700) -> (w698:dbl[])
                        n158 = Multiply(x=w697, y=w698) -> (x*y=w694:dbl[])
                        n159 = Add(x=w695, y=w694) -> (x+y=w696:dbl[])
                      }
                    }
                    n160 = Index Array(array=w683, index (row)=w684) -> (element=w674:dbl[])  [unwired: 1 in]
                    n161 = call "getPieceAngle.vi"("Center Num"=w674, "Center Piece"=w663) -> ("Angle"=w657:dbl)
                    n162 = call "getPieceAngle.vi"("Center Num"=w671, "Center Piece"=w664) -> ("Angle"=w658:dbl)
                    n163 = Add(x=1.5707963267948966, y=w649) -> (x+y=w648:dbl)
                    n164 = Round To Nearest(number=w663) -> (nearest integer value=w666:dbl[])
                    n165 = Round To Nearest(number=w664) -> (nearest integer value=w665:dbl[])
                    n166 = Add(x=1.5707963267948966, y=w648) -> (x+y=w647:dbl)
                    n167 = Subtract(x=w648, y=w658) -> (x-y=w650:dbl)
                    n168 = Subtract(x=w647, y=w657) -> (x-y=w653:dbl)
                    n169 = Greater?(x=w650, y=w649) -> (0:w655:bool)
                    n170 = Greater?(x=w653, y=w649) -> (0:w654:bool)
                    n171 = Subtract(x=w650, y=w649) -> (x-y=w651:dbl)
                    n172 = Subtract(x=w653, y=w649) -> (x-y=w652:dbl)
                    n173 = Select(t=w651, s=w655, f=w650) -> (s? t:f=w639:dbl)
                    n174 = Select(t=w652, s=w654, f=w653) -> (s? t:f=w642:dbl)
                    n175 = Subtract(x=w642, y=6.283185307179586) -> (x-y=w635:dbl)
                    n176 = Greater?(x=w642, y=w645) -> (0:w644:bool)
                    n177 = Subtract(x=w639, y=6.283185307179586) -> (x-y=w638:dbl)
                    n178 = Greater?(x=w639, y=w645) -> (0:w643:bool)
                    n179 = Select(t=w635, s=w644, f=w642) -> (s? t:f=w636:dbl)
                    n180 = Select(t=w638, s=w643, f=w639) -> (s? t:f=w637:dbl)
                    n181 = Multiply(x=w636, y=w667) -> (x*y=w660:dbl)
                    n182 = Multiply(x=w667, y=w637) -> (x*y=w659:dbl)
                    n183 = Round To Nearest(number=w660) -> (nearest integer value=w662:dbl)
                    n184 = Round To Nearest(number=w659) -> (nearest integer value=w661:dbl)
                  }
                  frame True {
                  }
                }
                "pick angle" <- w620
                "pick pos Norm" <- w628
                "place angle" <- w619
                "place pos Norm" <- w624
                n185 = Index Array(array=w628, index=0) -> (element=w623:dbl)
                n186 = Index Array(array=w628, index=1) -> (element=w616:dbl)
                n187 = Index Array(array=w624, index=0) -> (element=w618:dbl)
                n188 = Index Array(array=w624, index=1) -> (element=w617:dbl)
                n189 = Negate(x=w616) -> (-x=w615:dbl)
                "Passa Vez" <- w622
                "Dobrao" <- w621
              }
              frame #6 {
                n190 = shared-variable "My Computer\\Projeto_Modbus_Finalizado.lvlib\\000021"(TRUE ("000021")) -> ()  [unwired: 1 in, 1 out]
                n191 = Wait (ms)(milliseconds to wait=u32 1000) -> ()  [unwired: 1 out]
              }
              frame #7 {
                n192 = shared-variable "My Computer\\Projeto_Modbus_Finalizado.lvlib\\000021"(FALSE ("000021")) -> ()  [unwired: 1 in, 1 out]
              }
            }
          }
        }
        n193 = shared-variable "My Computer\\Projeto_Modbus_Finalizado.lvlib\\000018"(w355) -> ()  [unwired: 1 in, 1 out]
        n194 = shared-variable "My Computer\\Projeto_Modbus_Finalizado.lvlib\\000019"(w356) -> ()  [unwired: 1 in, 1 out]
        n195 = shared-variable "My Computer\\Projeto_Modbus_Finalizado.lvlib\\400130"(w353) -> ()  [unwired: 1 in, 1 out]
        n196 = shared-variable "My Computer\\Projeto_Modbus_Finalizado.lvlib\\400129"(w354) -> ()  [unwired: 1 in, 1 out]
        n197 = shared-variable "My Computer\\Projeto_Modbus_Finalizado.lvlib\\400133"(w352) -> ()  [unwired: 1 in, 1 out]
        n198 = shared-variable "My Computer\\Projeto_Modbus_Finalizado.lvlib\\400134"(w351) -> ()  [unwired: 1 in, 1 out]
        n199 = shared-variable "My Computer\\Projeto_Modbus_Finalizado.lvlib\\400131"(w350) -> ()  [unwired: 1 in, 1 out]
        n200 = shared-variable "My Computer\\Projeto_Modbus_Finalizado.lvlib\\400132"(w349) -> ()  [unwired: 1 in, 1 out]
      }
    }
    frame #6 {
      n201 = call "Imaq Dispose"("Image"=w735, "error in (no error)"=w736) -> ()  [unwired: 4 in, 1 out]
      n202 = call "Imaq Dispose"("Image"=w737, "error in (no error)"=w738) -> ()  [unwired: 4 in, 1 out]
      n203 = call <vilib>:"IMAQdx Close Camera.vi"("error in"=w739, "Session In"=w740) -> ("error out"=w734:errorcluster)  [unwired: 9 in]
      n204 = call-poly <vilib>:"Undeploy Libraries.vi"("library path"=w730) -> ("error out"=w732:errorcluster)  [unwired: 8 in]
      n205 = call <vilib>:"IMAQdx Close Camera.vi"("error in"=w734, "Session In"=w733) -> ()  [unwired: 9 in, 1 out]
      n206 = Merge Errors(w732) -> (→"Error Out":errorcluster)
    }
  }
